vi "Write Scalar ValueChange.vi"(8 "error in":errorcluster, 9 "Data":u8[](array[numeric]), 10 "Timestamp":u64, 11 "Ring buffer DVR in":refnum<data-value>) -> (0 "error out":errorcluster, 2 "Value changed?":bool, 3 "Ring buffer DVR out":refnum<data-value>)   [LabVIEW 2021, in "Ring Buffer Time Series Data.lvlib"]
uses:
  Ring Buffer Time Series Data.lvlib
  SubVIs/DVR data.ctl
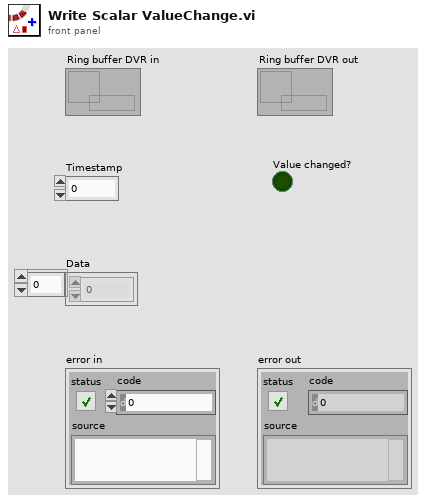
[diagram p1: front panel]
types:
  T1 = typedef "Ring Buffer Time Series Data.lvlib/DVR data.ctl" = cluster{"Timestamps":u64[], "Values":u8[], "#bytes per timestamp":i32, "Index":i32, "Size (#timestamps)":i32, "Full?":bool}
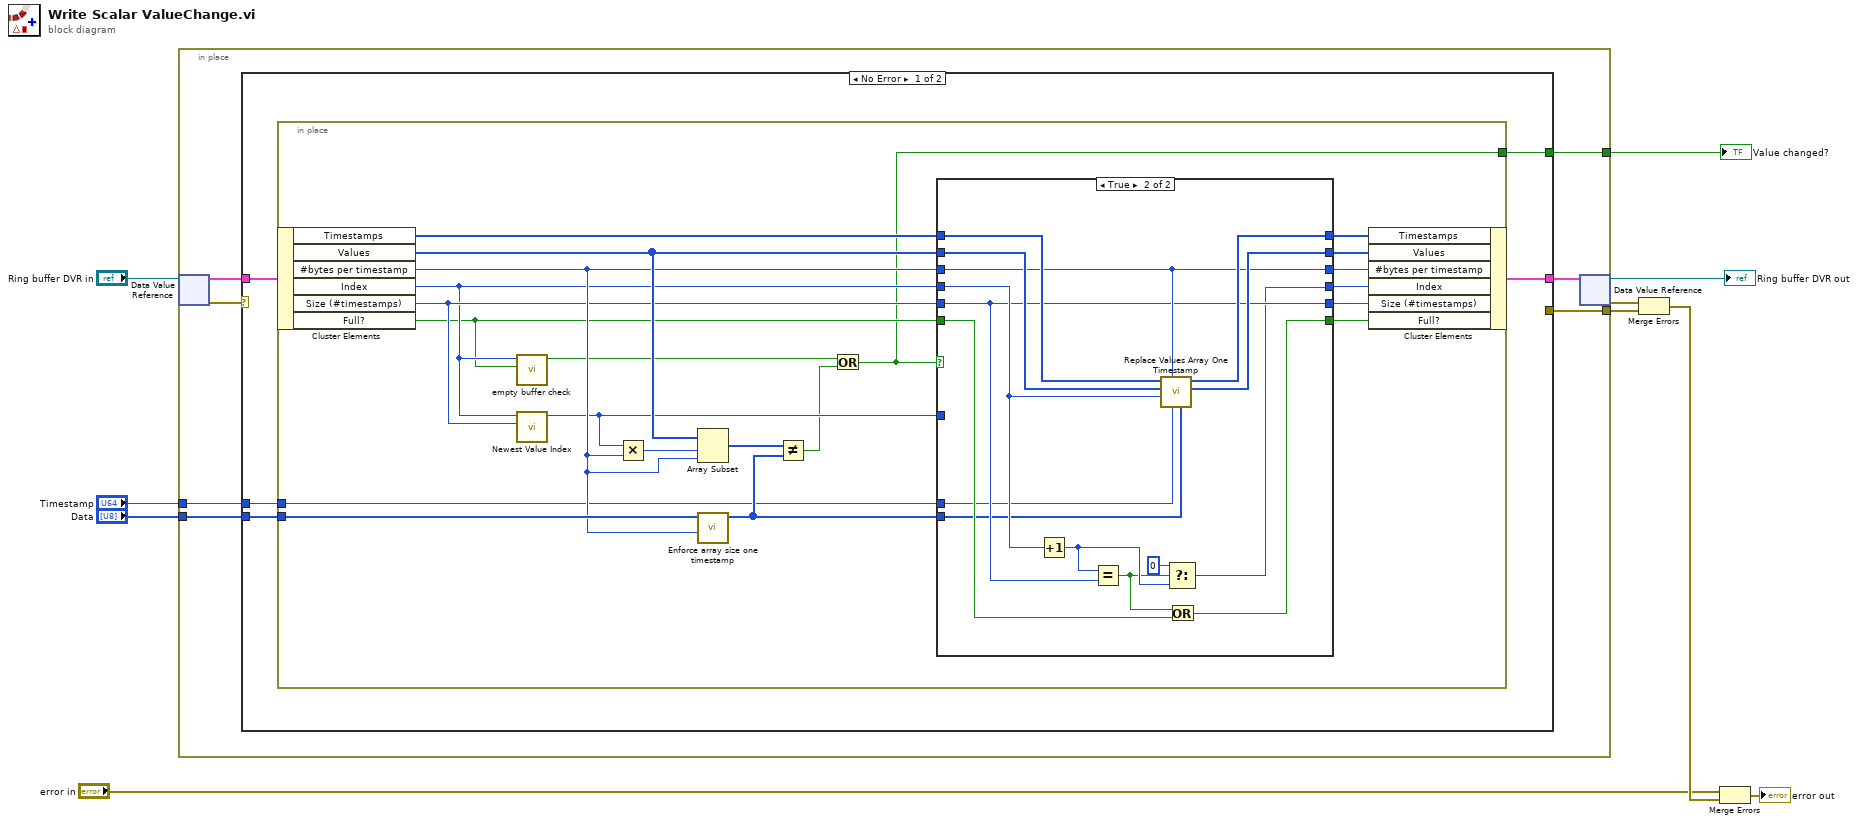
[diagram p0: block diagram]
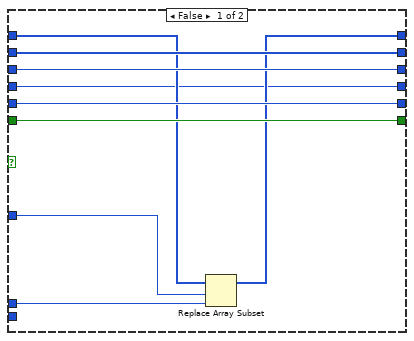
[diagram p2: hidden frame]
diagram:
  n1 = in-place {
    in-place-border: "Data" -> [w15]
    in-place-border: "Timestamp" -> [w14]
    in-place-border: [w12] -> w5
    in-place-border: [w11] -> w1
    n2 = in-place-dvr #1("Ring buffer DVR in") -> (w17:T1, w13:errorcluster)
    n3 = case shown="No Error" w13 {
      selector: w13 -> [_ w69]
      tunnel: w17 -> [w22 w68]
      tunnel: [w21 w68] -> w16
      tunnel: w15 -> [w20 _]
      tunnel: w14 -> [w19 _]
      tunnel: [_ w69] -> w12
      tunnel: [w18 _] -> w11
      frame No Error {
        n4 = in-place {
          in-place-border: w20 -> [w43]
          in-place-border: w19 -> [w31]
          in-place-border: [w23] -> w18
          n5 = in-place-cluster #2(w22) -> ("Timestamps"=w42:u64[], "Values"=w40:u8[], "#bytes per timestamp"=w38:i32, "Index"=w29:i32, "Size (#timestamps)"=w35:i32, "Full?"=w28:bool)
          n6 = call "empty buffer check.vi"("Full?"=w28, "Index"=w29) -> ("empty buffer?"=w25:bool)  [unwired: 9 in]
          n7 = call "Newest Value Index.vi"("Size"=w35, "Index"=w29) -> ("Newest value index"=w30:i32)  [unwired: 9 in]
          n8 = Multiply(x=w30, y=w38) -> (x*y=w27:i32)
          n9 = Array Subset(array=w40, index=w27, length=w38) -> (w26:u8[])
          n10 = call "Enforce array size one timestamp.vi"("#bytes per timestamp"=w38, "Values (new)"=w43) -> ("Values (new) [padded]"=w32:u8[])  [unwired: 9 in]
          n11 = Not Equal?(x=w26, y=w32) -> (x != y?=w24:bool)
          n12 = Or(x=w25, y=w24) -> (x .or. y?=w23:bool)
          n13 = case shown="True" w23 {
            tunnel: w42 -> [w48 w64]
            tunnel: [w47 w60] -> w41
            tunnel: w40 -> [w52 w63]
            tunnel: [w52 w59] -> w39
            tunnel: w38 -> [w51 w58]
            tunnel: [w51 w58] -> w37
            tunnel: w29 -> [w45 w62]
            tunnel: [w45 w56] -> w36
            tunnel: w35 -> [w50 w57]
            tunnel: [w50 w57] -> w34
            tunnel: w28 -> [w49 w61]
            tunnel: [w49 w55] -> w33
            tunnel: w32 -> [_ w54]
            tunnel: w31 -> [w46 w53]
            tunnel: w30 -> [w44 _]
            frame False {
              n14 = Replace Array Subset(array=w48, new element=w46, index=w44) -> (w47:u64[])
            }
            frame True {
              n15 = Increment(x=w62) -> (x+1=w67:i32)
              n16 = Equal?(x=w67, y=w57) -> (x = y?=w65:bool)
              n17 = call "Replace Values Array One Timestamp.vi"("Values (new)"=w54, "Timestamps (new)"=w53, "#bytes per timestamp"=w58, "index"=w62, "Values (buffered)"=w63, "Timestamps (buffered)"=w64) -> ("Values (buffered)"=w59:u8[], "Timestamps (buffered)"=w60:u64[])  [unwired: 4 in]
              n18 = Select(t=0, s=w65, f=w67) -> (s? t:f=w56:i32)
              n19 = Or(x=w65, y=w61) -> (x .or. y?=w55:bool)
            }
          }
          n20 = in-place-cluster #2("Timestamps"=w41, "Values"=w39, "#bytes per timestamp"=w37, "Index"=w36, "Size (#timestamps)"=w34, "Full?"=w33) -> (w21:T1)
        }
      }
      frame Error {
      }
    }
    n21 = in-place-dvr #1(w16) -> (→"Ring buffer DVR out":refnum<data-value>, w6:errorcluster)
  }
  "Value changed?" <- w1
  n22 = Merge Errors(w6, w5) -> (w4:errorcluster)
  n23 = Merge Errors("error in", w4) -> (→"error out":errorcluster)
